vi "Init.vi"(10 "Event jettl":refnum<class "Event jettl.lvclass">) -> (3 "Event Last Ack Msg Strategy out":refnum<class "Event Last Ack Msg Strategy.lvclass">)   [LabVIEW 2021, in "jettl.lvlib" / "Event Last Ack.lvlib" / "Event Last Ack Msg Strategy.lvclass"]
uses:
  Event Last Ack Msg Strategy.lvclass
  Event jettl/Event jettl.lvclass
  Event Last Ack Msg Strategy.lvclass/Event Last Ack Msg Strategy.ctl
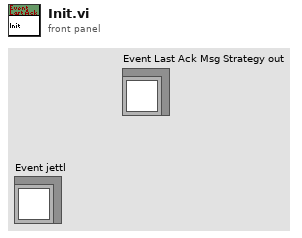
[diagram p1: front panel]
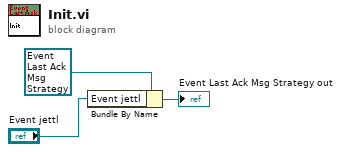
[diagram p0: block diagram]
diagram:
  n1 = Bundle By Name(cluster=refnum<class "Event Last Ack Msg Strategy.lvclass"> refnum ("Event Last Ack Msg out"), "Event jettl"="Event jettl") -> (→"Event Last Ack Msg Strategy out":refnum<class "Event Last Ack Msg Strategy.lvclass">)
